vi "HS_ReadCamera.vi"(8 "error in":errorcluster, 9 "Console In":string, 11 "VISA Refnum in":refnum<visa-resource-name>) -> (0 "error out":errorcluster, 1 "Console Out":string, 2 "Good?":bool, 3 "VISA Refnum out":refnum<visa-resource-name>, 4 "image data":T1, 5 "new picture":picture, 6 "length":i32, 7 "size()":u32[](array[numeric]))   [LabVIEW 2016]
uses:
  <vilib>/picture/picture.llb/imagedata.ctl
panel:
  out "read buffer":string
  # "23584"
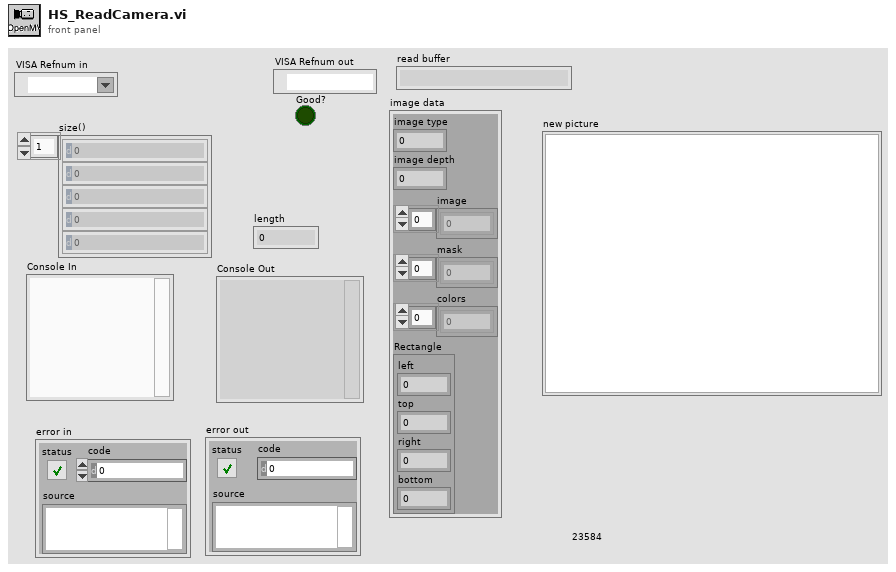
[diagram p1: front panel]
types:
  T1 = typedef "imagedata.ctl" = cluster{"image type":i32, "image depth":i32, "image":u8[], "mask":u8[], "colors":u32[], "Rectangle":cluster{"left":i16, "top":i16, "right":i16, "bottom":i16}}
  T2 = cluster{"Before":u8, "After":u8, "Send as 1 block?":bool}
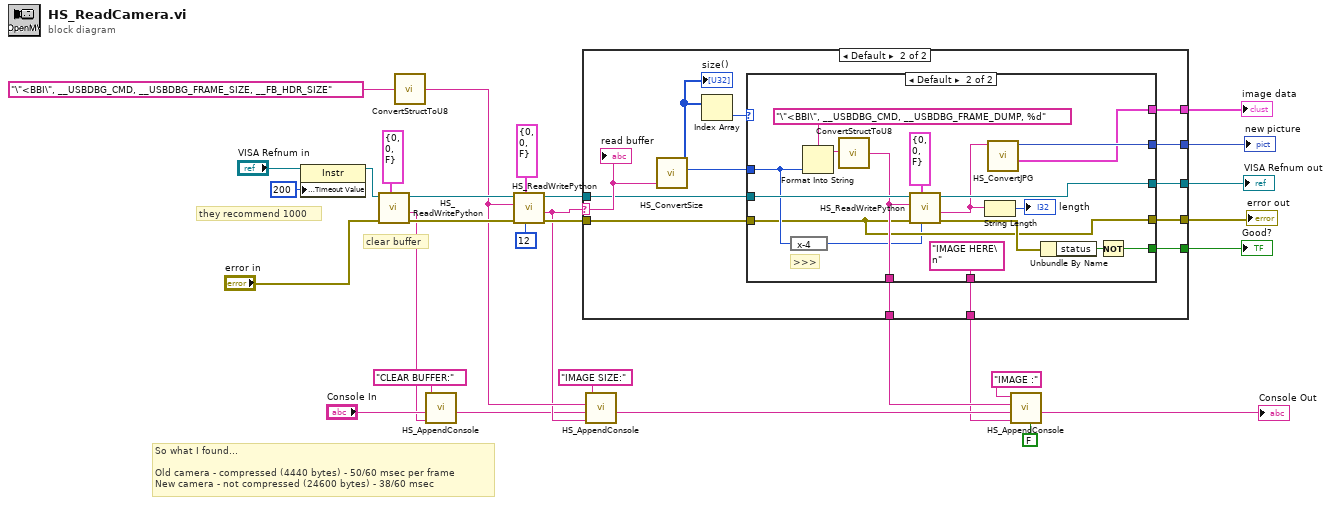
[diagram p0: block diagram]
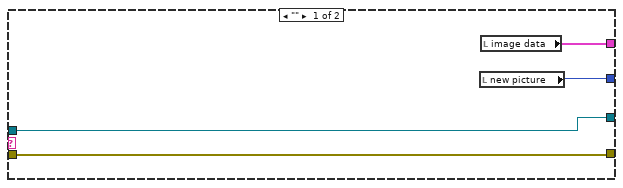
[diagram p2: hidden frame]
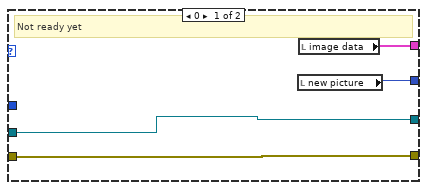
[diagram p3: hidden frame]
diagram:
  # "they recommend 1000"
  # "So what I found...\n\nOld camera - compressed (4440 bytes) - 50/60 msec per frame\nNew camera - not compressed (24600 bytes) - 38/60 msec"
  # "clear buffer"
  n1 = property class="Instr"(reference="VISA Refnum in", "General Settings:Timeout Value"=u32 200) -> (reference out=w19:refnum<visa-resource-name>)  [unwired: 1 in, 1 out]
  n2 = call <userlib>:"HS_ReadWritePython.vi"("Timeouts (ms)"=T2 {"Before"=0, "After"=0, "Send as 1 block?"=FALSE}, "error in"="error in", "VISA in"=w19) -> ("error out"=w16:errorcluster, "Console Out"=w5:string, "VISA out"=w18:refnum<visa-resource-name>)  [unwired: 3 in, 3 out]
  n3 = call <userlib>:"ConvertStructToU8.vi"("struct"="\"<BBI\", __USBDBG_CMD, __USBDBG_FRAME_SIZE, __FB_HDR_SIZE" ("write buffer")) -> ("Binary"=w14:string)
  n4 = call <userlib>:"HS_AppendConsole.vi"("Reply"=w5, "Console in"="Console In", "Command"="CLEAR BUFFER:") -> ("Console Out"=w4:string)  [unwired: 8 in]
  n5 = call <userlib>:"HS_ReadWritePython.vi"("Reply length"=12, "Timeouts (ms)"=T2 {"Before"=0, "After"=0, "Send as 1 block?"=FALSE}, "error in"=w16, "Write"=w14, "VISA in"=w18) -> ("error out"=w22:errorcluster, "Console Out"=w13:string, "VISA out"=w21:refnum<visa-resource-name>)  [unwired: 1 in, 3 out]
  n6 = case shown="Default" w13 {
    selector: w13 -> [_ w39]
    tunnel: [w34 w47] -> w30
    tunnel: [w33 w46] -> w23
    tunnel: w21 -> [w34 w37]
    tunnel: w22 -> [w33 w43]
    tunnel: [w31 w42] -> w28
    tunnel: [w32 w41] -> w27
    tunnel: [_ w40] -> w26
    tunnel: [_ w36] -> w9
    tunnel: [_ w35] -> w11
    frame "" {
      n7 = local read "new picture"() -> (w31:picture)
      n8 = local read "image data"() -> (w32:T1)
    }
    frame Default {
      n9 = call <userlib>:"HS_ConvertSize.vi"("read buffer"=w39) -> ("# bytes"=w45:u32, "size()"=w38:u32[])  [unwired: 9 in]
      "size()" <- w38
      n10 = Index Array(array=w38) -> (element=w44:u32)  [unwired: 1 in]
      n11 = case shown="Default" w44 {
        tunnel: [w50 w60] -> w47
        tunnel: [w51 w53] -> w46
        tunnel: w45 -> [_ w61]
        tunnel: w37 -> [w50 w62]
        tunnel: w43 -> [w51 w53]
        tunnel: [w49 w66] -> w42
        tunnel: [w48 w65] -> w41
        tunnel: [_ w63] -> w40
        tunnel: [_ "IMAGE HERE\n"] -> w36
        tunnel: [_ w57] -> w35
        frame 0 {
          # "Not ready yet"
          n12 = local read "new picture"() -> (w49:picture)
          n13 = local read "image data"() -> (w48:T1)
        }
        frame Default {
          # ">>>"
          n14 = expression code="x-4"(w61) -> (w52:u32)
          n15 = Format Into String(format string="\"<BBI\", __USBDBG_CMD, __USBDBG_FRAME_DUMP, %d" ("write buffer"), w61) -> (resulting string=w67:string)  [unwired: 2 in, 1 out]
          n16 = call <userlib>:"ConvertStructToU8.vi"("struct"=w67) -> ("Binary"=w57:string)
          n17 = call <userlib>:"HS_ReadWritePython.vi"("Reply length"=w52, "Timeouts (ms)"=T2 {"Before"=0, "After"=0, "Send as 1 block?"=FALSE}, "error in"=w53, "Write"=w57, "VISA in"=w62) -> ("error out"=w59:errorcluster, "Console Out"=w55:string, "VISA out"=w60:refnum<visa-resource-name>)  [unwired: 1 in, 3 out]
          n18 = String Length(string=w55) -> (length=→"length":i32)
          n19 = call <userlib>:"HS_ConvertJPG.vi"("buffer"=w55) -> ("image data"=w65:T1, "new picture"=w66:picture)  [unwired: 9 in]
          n20 = Unbundle By Name(w59) -> ("status"=w64:bool)
          n21 = Not(x=w64) -> (.not. x?=w63:bool)
        }
      }
      "read buffer" <- w39
    }
  }
  "VISA Refnum out" <- w30
  "error out" <- w23
  "new picture" <- w28
  "image data" <- w27
  "Good?" <- w26
  n22 = call <userlib>:"HS_AppendConsole.vi"("Reply"=w13, "Console in"=w4, "Send"=w14, "Command"="IMAGE SIZE:") -> ("Console Out"=w10:string)  [unwired: 7 in]
  n23 = call <userlib>:"HS_AppendConsole.vi"("Show Reply Binary?"=FALSE ("Show Send Binary?"), "Reply"=w9, "Console in"=w10, "Send"=w11, "Command"="IMAGE :") -> ("Console Out"=→"Console Out":string)  [unwired: 6 in]
